vi "Generate Client.vi"(8 "error in":errorcluster, 9 "client name":string, 10 "service class":string, 11 "project path":path) -> (0 "error out":errorcluster)   [LabVIEW 2021, in "NI Measurement V2 Client Generator Runtime.lvlib"]
doc: "Generates client for the measurement plug-in referred by the service class."
uses:
  NI Measurement V2 Client Generator Runtime.lvlib
  Client Generator Error Strings Global.vi
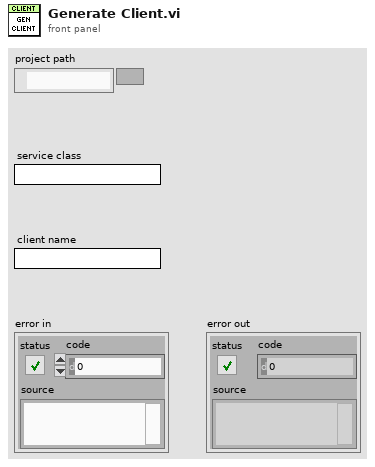
[diagram p1: front panel]
types:
  T1 = typedef "Measurement Service Client V2.lvlib/ni_measurementlink_measurement_v2_GetMetadataResponse.ctl" = cluster{"measurement_details":T2, "measurement_signature":T3, "user_interface_details":T10[]}
  T2 = typedef "Measurement Service Client V2.lvlib/ni_measurementlink_measurement_v2_MeasurementDetails.ctl" = cluster{"display_name":string, "version":string}
  T3 = typedef "Measurement Service Client V2.lvlib/ni_measurementlink_measurement_v2_MeasurementSignature.ctl" = cluster{"configuration_parameters_message_type":string, "configuration_parameters":T4[], "configuration_defaults":T7, "outputs_message_type":string, "outputs":T8[]}
  T4 = typedef "Measurement Service Client V2.lvlib/ni_measurementlink_measurement_v2_ConfigurationParameter.ctl" = cluster{"field_number":i32, "type":T5, "name":string, "repeated":bool, "annotations":T6[], "message_type":string}
  T5 = typedef "Measurement Service Client V2.lvlib/google_protobuf_Field_Kind.ctl" = enum32{"TYPE_UNKNOWN", "TYPE_DOUBLE", "TYPE_FLOAT", "TYPE_INT64", "TYPE_UINT64", "TYPE_INT32", "TYPE_FIXED64", "TYPE_FIXED32", "TYPE_BOOL", "TYPE_STRING", "TYPE_GROUP", "TYPE_MESSAGE", "TYPE_BYTES", "TYPE_UINT32", "TYPE_ENUM", "TYPE_SFIXED32", "TYPE_SFIXED64", "TYPE_SINT32", "TYPE_SINT64"}
  T6 = typedef "Measurement Service Client V2.lvlib/ni_measurementlink_measurement_v2_ConfigurationParameter_AnnotationsEntry.ctl" = cluster{"key":string, "value":string}
  T7 = typedef "Measurement Service Client V2.lvlib/google_protobuf_Any.ctl" = cluster{"type_url":string, "value":u8[]}
  T8 = typedef "Measurement Service Client V2.lvlib/ni_measurementlink_measurement_v2_Output.ctl" = cluster{"field_number":i32, "type":T5, "name":string, "repeated":bool, "annotations":T9[], "message_type":string}
  T9 = typedef "Measurement Service Client V2.lvlib/ni_measurementlink_measurement_v2_Output_AnnotationsEntry.ctl" = cluster{"key":string, "value":string}
  T10 = typedef "Measurement Service Client V2.lvlib/ni_measurementlink_measurement_v2_UserInterfaceDetails.ctl" = cluster{"file_url":string}
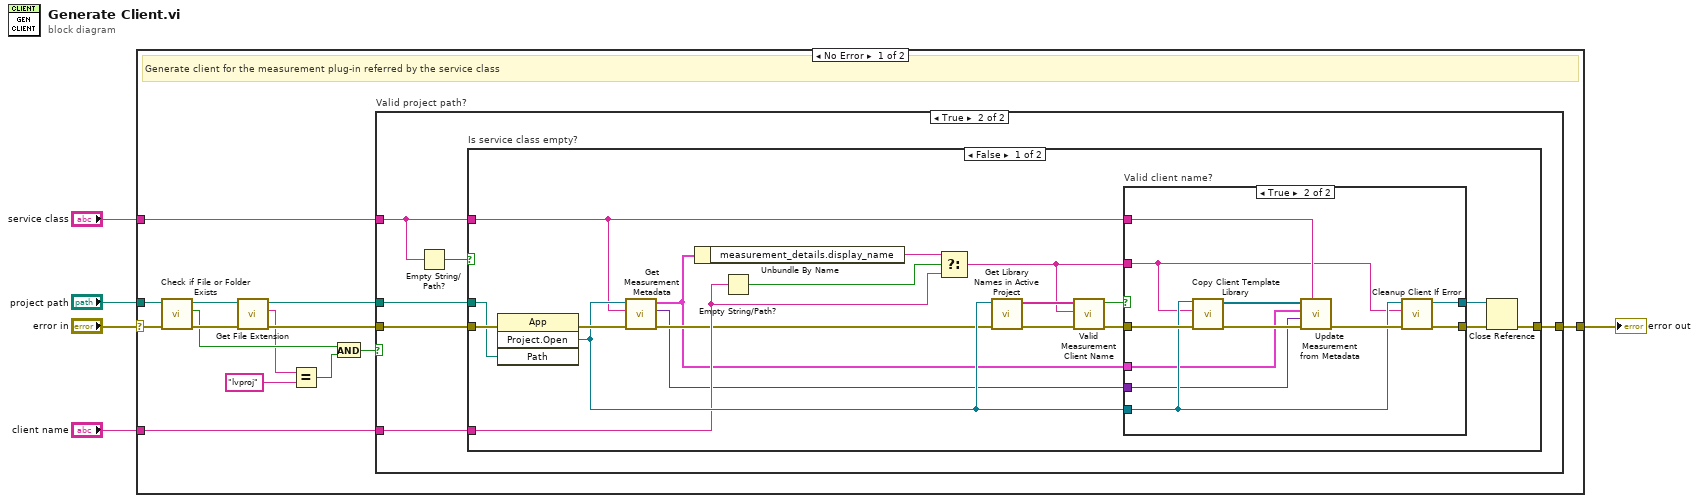
[diagram p0: block diagram]
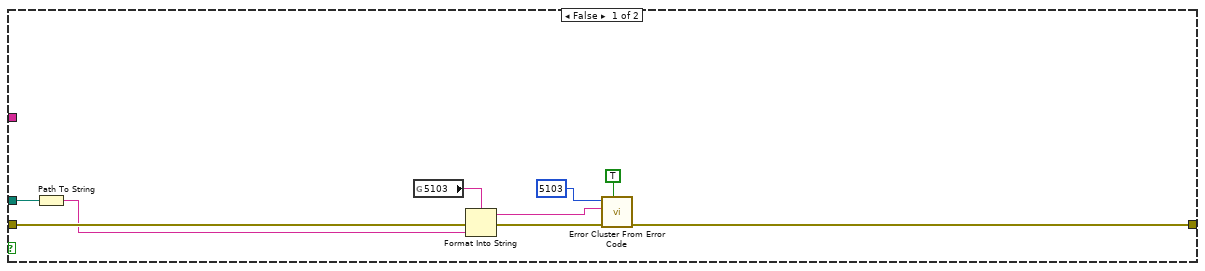
[diagram p2: hidden frame]
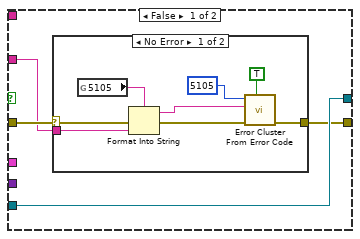
[diagram p3: hidden frame]
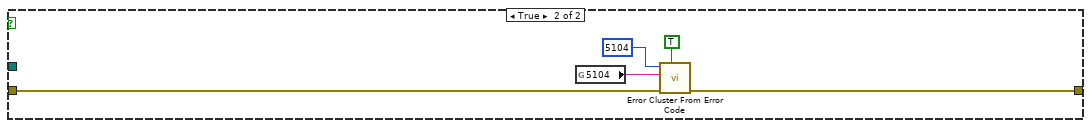
[diagram p5: hidden frame]
diagram:
  n1 = case shown="No Error" "error in" {
    selector: "error in" -> [w18 w83]
    tunnel: "service class" -> [w19 _]
    tunnel: [w6 w83] -> w1
    tunnel: "project path" -> [w15 _]
    tunnel: "client name" -> [w7 _]
    frame No Error {
      # "Generate client for the measurement plug-in referred by the service class"
      n2 = call <vilib>:"Check if File or Folder Exists.vi"("error in (no error)"=w18, "path"=w15) -> ("error out"=w17:errorcluster, "file or folder exists?"=w14:bool, "dup path"=w13:path)  [unwired: 7 in]
      n3 = call <vilib>:"Get File Extension.vi"("error in (no error)"=w17, "file"=w13) -> ("error out"=w16:errorcluster, "lowercase file extension"=w9:string, "dup file"=w12:path)  [unwired: 5 in, 2 out]
      n4 = Equal?(x=w9, y="lvproj") -> (x = y?=w8:bool)
      n5 = And(x=w14, y=w8) -> (x .and. y?=w11:bool)
      n6 = case "Valid project path?" shown="True" w11 {
        tunnel: w19 -> [_ w30]
        tunnel: [w27 w32] -> w6
        tunnel: w16 -> [w28 w34]
        tunnel: w12 -> [w20 w33]
        tunnel: w7 -> [_ w31]
        frame False {
          n7 = Path To String(path=w20) -> (string=w22:string)
          n8 = global read "Client Generator Error Strings Global.vi" "5103"() -> (w23:string)
          n9 = Format Into String(format string=w23, error in=w28, w22) -> (resulting string=w21:string, error out=w24:errorcluster)  [unwired: 1 in]
          n10 = call <vilib>:"Error Cluster From Error Code.vi"("show call chain? (False)"=TRUE, "error in (no error)"=w24, "error message (\"\")"=w21, "error code (0)"=5103) -> ("error out"=w27:errorcluster)  [unwired: 5 in]
        }
        frame True {
          n11 = Empty String/Path?(string/path=w30) -> (empty?=w29:bool)
          n12 = case "Is service class empty?" shown="False" w29 {
            tunnel: w34 -> [w53 w82]
            tunnel: w33 -> [w52 _]
            tunnel: [w36 w81] -> w32
            tunnel: w31 -> [w49 _]
            tunnel: w30 -> [w38 _]
            frame False {
              n13 = invoke class="App" method="Project.Open"(error in=w53, "Path"=w52) -> (error out=w51:errorcluster, "Project:Open"=w50:refnum<vi>)  [unwired: 2 in, 2 out]
              n14 = call "Get Measurement Metadata.vi"("error in"=w51, "service_class"=w38, "project refnum"=w50) -> ("error out"=w45:errorcluster, "default value"=w40:variant, "metadata"=w41:T1)  [unwired: 6 in]
              n15 = Unbundle By Name(w41) -> ("measurement_details.display_name"=w43:string)
              n16 = Empty String/Path?(string/path=w49) -> (empty?=w44:bool)
              n17 = Select(t=w43, s=w44, f=w49) -> (s? t:f=w42:string)
              n18 = call "Get Library Names in Active Project.vi"("error in (no error)"=w45, "project ref"=w50) -> ("error out"=w48:errorcluster, "library names"=w46:string[])  [unwired: 8 in]
              n19 = call "Valid Measurement Client Name.vi"("error in"=w48, "requested client name"=w42, "library names"=w46) -> ("error out"=w47:errorcluster, "valid name?"=w39:bool)  [unwired: 7 in]
              n20 = case "Valid client name?" shown="True" w39 {
                tunnel: [w57 w67] -> w35
                tunnel: [w55 w74] -> w37
                tunnel: w47 -> [w56 w72]
                tunnel: w38 -> [_ w73]
                tunnel: w50 -> [w57 w71]
                tunnel: w41 -> [_ w69]
                tunnel: w40 -> [_ w68]
                tunnel: w42 -> [w54 w70]
                frame False {
                  n21 = case shown="No Error" w56 {
                    selector: w56 -> [w65 w66]
                    tunnel: [w64 w66] -> w55
                    tunnel: w54 -> [w59 _]
                    frame No Error {
                      n22 = global read "Client Generator Error Strings Global.vi" "5105"() -> (w60:string)
                      n23 = Format Into String(format string=w60, error in=w65, w59) -> (resulting string=w61:string, error out=w63:errorcluster)  [unwired: 1 in]
                      n24 = call <vilib>:"Error Cluster From Error Code.vi"("show call chain? (False)"=TRUE, "error in (no error)"=w63, "error message (\"\")"=w61, "error code (0)"=5105) -> ("error out"=w64:errorcluster)  [unwired: 5 in]
                    }
                    frame Error {
                    }
                  }
                }
                frame True {
                  n25 = call "Copy Client Template Library.vi"("error in"=w72, "new library name"=w70, "project ref"=w71) -> ("error out"=w77:errorcluster, "file refnums"=w75:refnum<vi>[])  [unwired: 7 in]
                  n26 = call "Update Measurement from Metadata.vi"("client service_class"=w73, "error in"=w77, "default value"=w68, "metadata"=w69, "file refnums"=w75) -> ("error out"=w76:errorcluster)  [unwired: 6 in]
                  n27 = call "Cleanup Client If Error.vi"("error in"=w76, "client name"=w70, "project ref in"=w71) -> ("error out"=w74:errorcluster, "project ref out"=w67:refnum<vi>)  [unwired: 7 in]
                }
              }
              n28 = Close Reference(reference=w35, error in (no error)=w37) -> (error out=w36:errorcluster)
            }
            frame True {
              n29 = global read "Client Generator Error Strings Global.vi" "5104"() -> (w78:string)
              n30 = call <vilib>:"Error Cluster From Error Code.vi"("show call chain? (False)"=TRUE, "error in (no error)"=w82, "error message (\"\")"=w78, "error code (0)"=5104) -> ("error out"=w81:errorcluster)  [unwired: 5 in]
            }
          }
        }
      }
    }
    frame Error {
      # "Pass"
    }
  }
  "error out" <- w1
